vi "callback_range_call.vi"(5 "Attribute Value":dbl format="%_6g", 7 "Attribute":T1={"Identifier"="", "Descriptive name"="", "Data Type"=enum."Integer 32", "Command"="", "Access"=2, "Range Table"="", "Read Callback"="", "Write Callback"="", "Range Callback"="", "Check Callback"="", "Rngtable Callback"="", "Coerce Callback"="", "Supported Models"="", "Instrument Options"="", "Repeated Capabilities"="", "Check Status Callback"="", "Index"=0, "Flag: OPC Wait"=FALSE, "Flag: Dont check status"=FALSE, "Flag: Cache Only"=FALSE} {"Access" items=["Read Only", "Write Only", "Read/Write"]}, 8 "error in":errorcluster, 11 "VISA resource name":refnum<visa-resource-name>) -> (0 "error out":errorcluster, 1 "Enum output":string, 2 "Enum?":bool, 3 "VISA resource name out":refnum<visa-resource-name>)   [LabVIEW 2014, in "rszvl_rsidr_core.lvlib"]
uses:
  rszvl_rsidr_core.lvlib
  type_Attribute.ctl
  type_Attribute_Data_Type.ctl
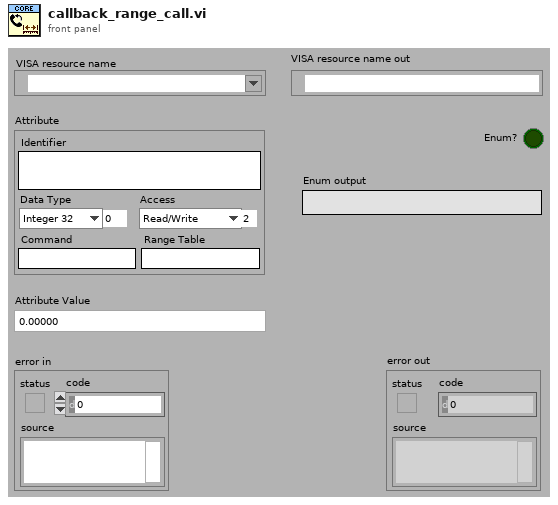
[diagram p1: front panel]
types:
  T1 = typedef "rszvl_rsidr_core.lvlib/type_Attribute.ctl" = cluster{"Identifier":string, "Descriptive name":string, "Data Type":T2, "Command":string, "Access":u16, "Range Table":string, "Read Callback":string, "Write Callback":string, "Range Callback":string, "Check Callback":string, "Rngtable Callback":string, "Coerce Callback":string, "Supported Models":string, "Instrument Options":string, "Repeated Capabilities":string, "Check Status Callback":string, "Index":i32, "Flag: OPC Wait":bool, "Flag: Dont check status":bool, "Flag: Cache Only":bool}
  T2 = typedef "rszvl_rsidr_core.lvlib/type_Attribute_Data_Type.ctl" = enum16{"Integer 32", "Double", "String", "Boolean", "None", "Integer 64"}
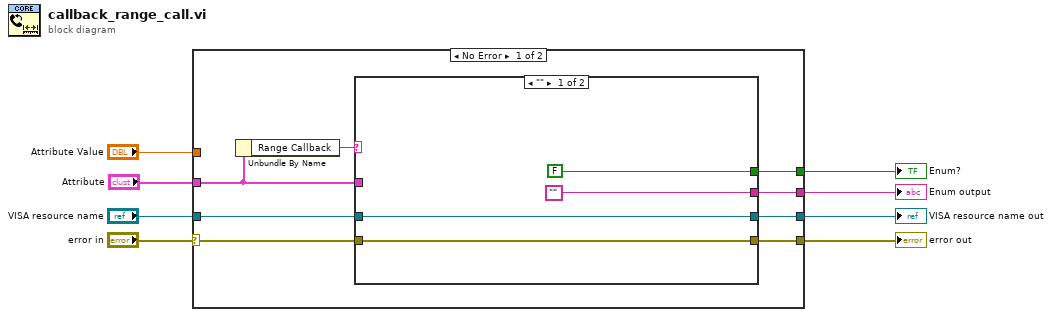
[diagram p0: block diagram]
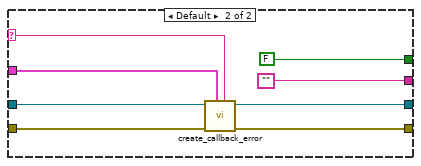
[diagram p2: hidden frame]
diagram:
  n1 = case shown="No Error" "error in" {
    selector: "error in" -> [w12 w29]
    tunnel: [w13 w29] -> w4
    tunnel: "VISA resource name" -> [w15 w30]
    tunnel: [w14 w30] -> w3
    tunnel: "Attribute" -> [w9 _]
    tunnel: "Attribute Value" -> [_ _]
    tunnel: [w11 _] -> w2
    tunnel: [w10 _] -> w1
    frame No Error {
      n2 = Unbundle By Name(w9) -> ("Range Callback"=w16:string)
      n3 = case shown="\"\"" w16 {
        selector: w16 -> [_ w23]
        tunnel: w15 -> [w20 w27]
        tunnel: [w20 w25] -> w14
        tunnel: [w19 w26] -> w13
        tunnel: w12 -> [w19 w28]
        tunnel: ["" ("Empty String Constant") "" ("Empty String Constant")] -> w11
        tunnel: [FALSE FALSE] -> w10
        tunnel: w9 -> [_ w24]
        frame "" {
        }
        frame Default {
          n4 = call "create_callback_error.vi"("Callback Name"=w23, "Attribute"=w24, "error in"=w28, "VISA resource name"=w27) -> ("error out"=w26:errorcluster, "VISA resource name out"=w25:refnum<visa-resource-name>)  [unwired: 6 in]
        }
      }
    }
    frame Error {
    }
  }
  "error out" <- w4
  "VISA resource name out" <- w3
  "Enum output" <- w2
  "Enum?" <- w1
